vi "HardwareLogLoop.vi"(8 "Error In":errorcluster, 9 "ABLE Configuration":T1, 10 "Hardware Log Data":refnum<queue>, 11 "Hardware Log Action Queue":refnum<queue>) -> (0 "Error Out":errorcluster)   [LabVIEW 2012]
uses:
  ABLEConfiguration.ctl
  DisplayConfiguration.ctl
  FolderConfiguration.ctl
  AlarmsConfiguration.ctl
  Keithley6485Configuration.ctl
  Keithley6482Configuration.ctl
  HardwareLogActionQueueElement.ctl
  HardwareLogAction.ctl
  HardwareLogData.ctl
  HardwareDisplayData.ctl
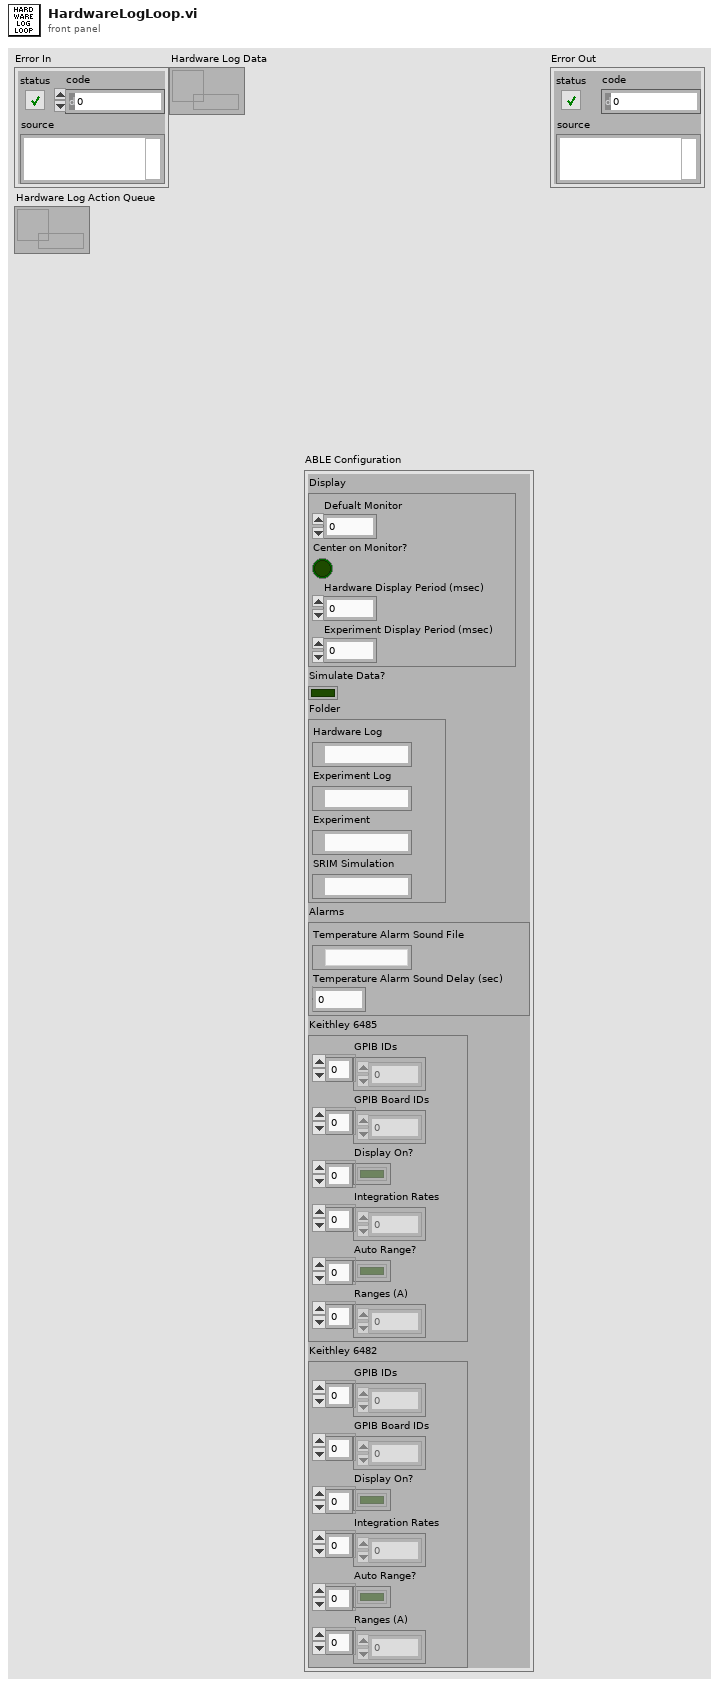
[diagram p1: front panel]
types:
  T1 = typedef "ABLEConfiguration.ctl" = cluster{"Display":T2, "Simulate Data?":bool, "Folder":T3, "Alarms":T4, "Keithley 6485":T5, "Keithley 6482":T6}
  T2 = typedef "DisplayConfiguration.ctl" = cluster{"Defualt Monitor":u16, "Center on Monitor?":bool, "Hardware Display Period (msec)":u32, "Experiment Display Period (msec)":u32}
  T3 = typedef "FolderConfiguration.ctl" = cluster{"Hardware Log":path, "Experiment Log":path, "Experiment":path, "SRIM Simulation":path}
  T4 = typedef "AlarmsConfiguration.ctl" = cluster{"Temperature Alarm Sound File":path, "Temperature Alarm Sound Delay (sec)":dbl}
  T5 = typedef "Keithley6485Configuration.ctl" = cluster{"GPIB IDs":u8[], "GPIB Board IDs":u8[], "Display On?":bool[], "Integration Rates":dbl[], "Auto Range?":bool[], "Ranges (A)":dbl[]}
  T6 = typedef "Keithley6482Configuration.ctl" = cluster{"GPIB IDs":u8[], "GPIB Board IDs":u8[], "Display On?":bool[], "Integration Rates":dbl[], "Auto Range?":bool[], "Ranges (A)":dbl[]}
  T7 = typedef "HardwareLogActionQueueElement.ctl" = cluster{"Action":T8, "Data":variant}
  T8 = typedef "HardwareLogAction.ctl" = enum16{"Initialize", "Clear", "Create", "Log", "Stop", "Shutdown"}
  T9 = enum16{"open", "replace", "create", "open or create", "replace or create", "replace or create with confirmation"}
  T10 = typedef "HardwareLogData.ctl" = cluster{"Time Stamp":timestamp, "Data":T11}
  T11 = typedef "HardwareDisplayData.ctl" = cluster{"Temperatures (C)":dbl[], "Terminal Voltage (MeV)":dbl, "Currents (A)":dbl[]}
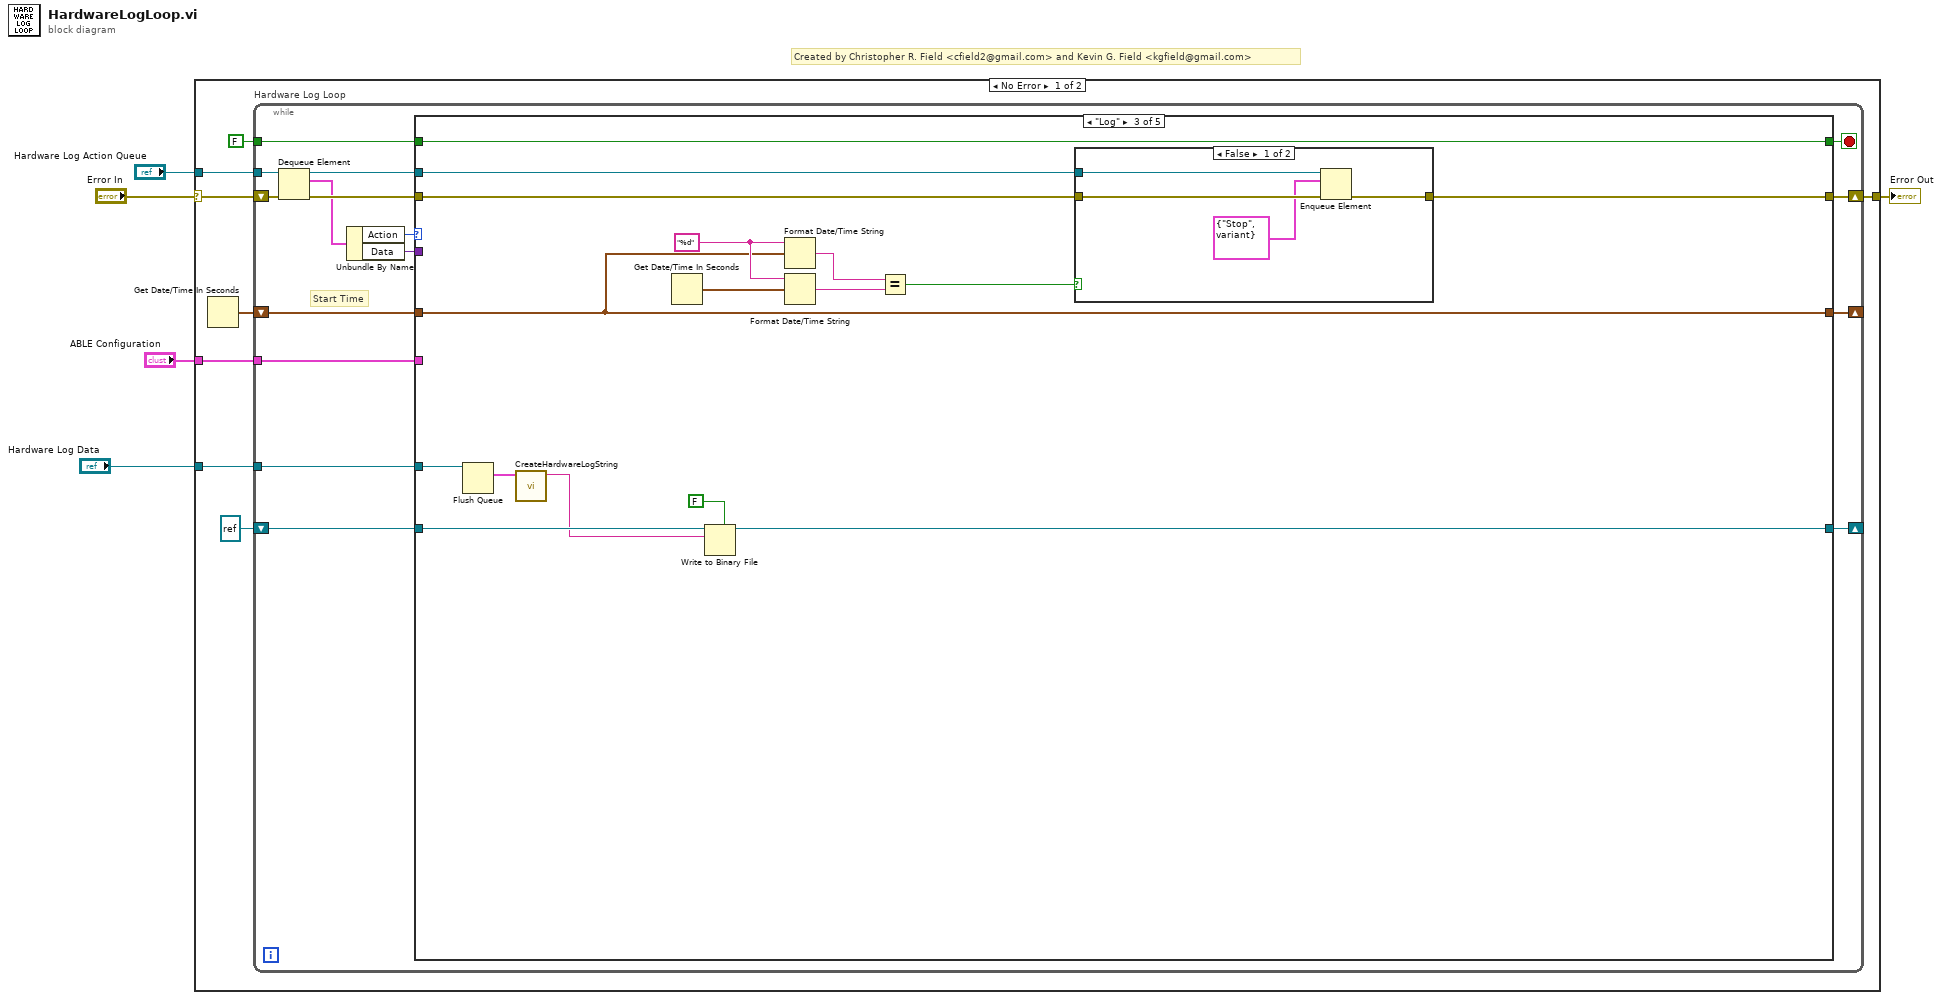
[diagram p0: block diagram]
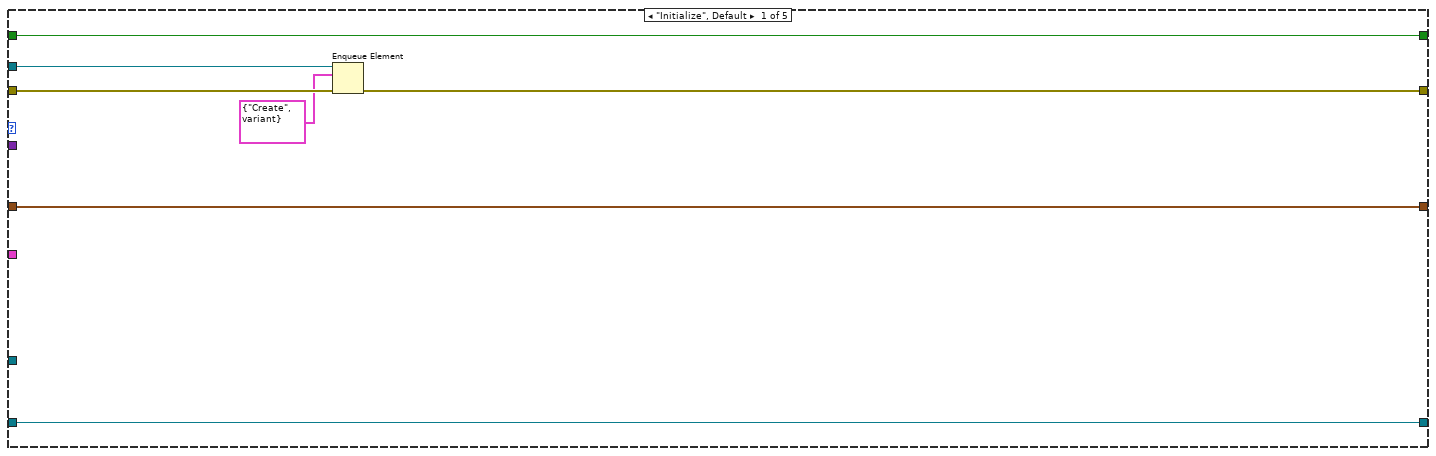
[diagram p2: hidden frame]
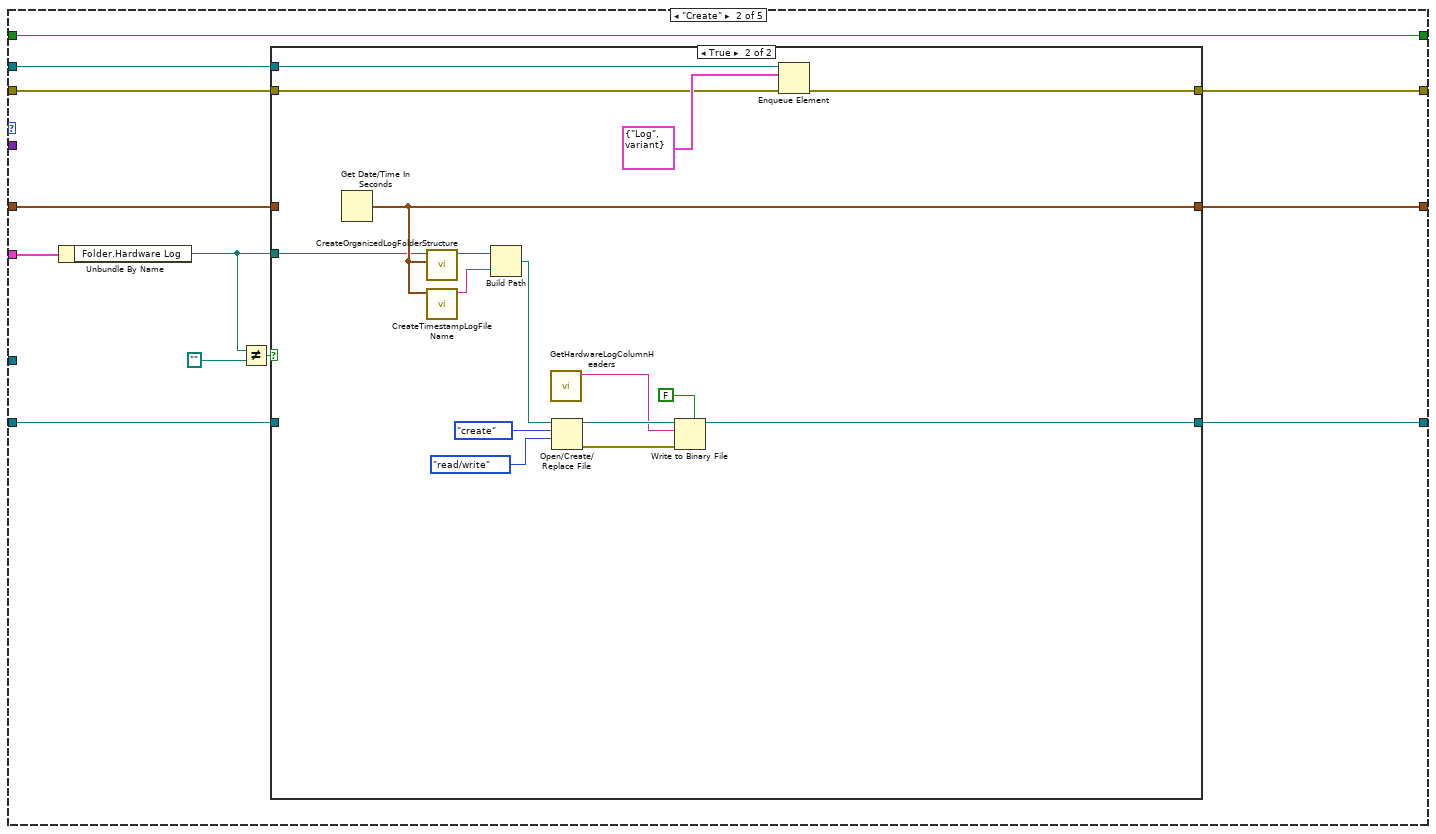
[diagram p3: hidden frame]
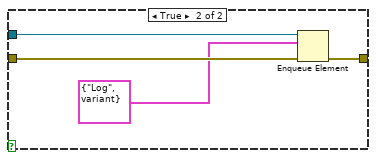
[diagram p5: hidden frame]
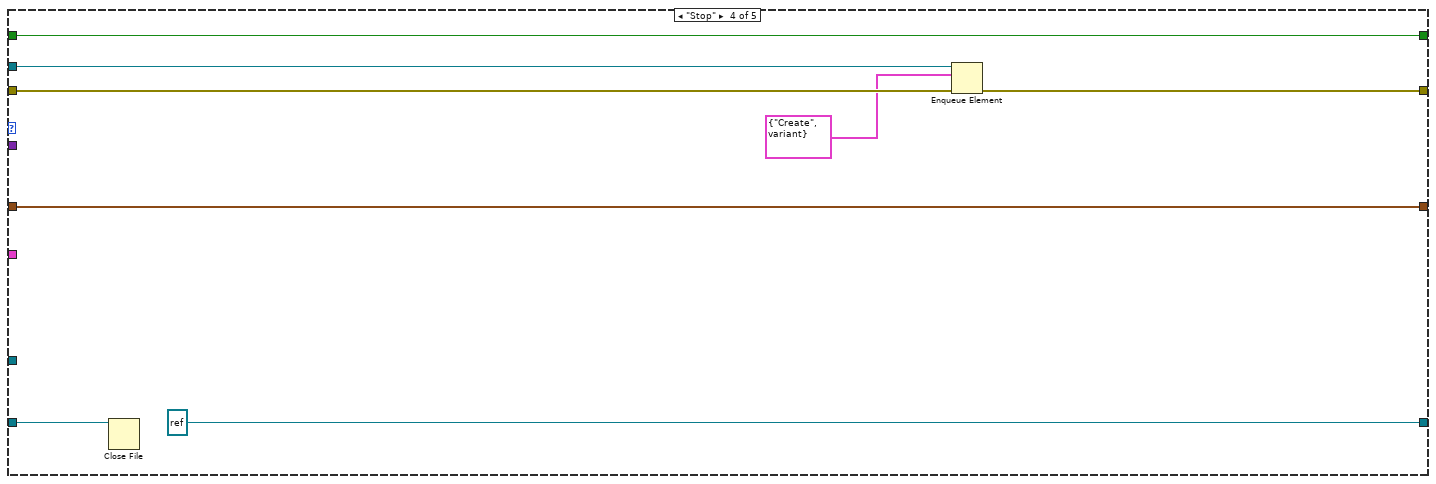
[diagram p6: hidden frame]
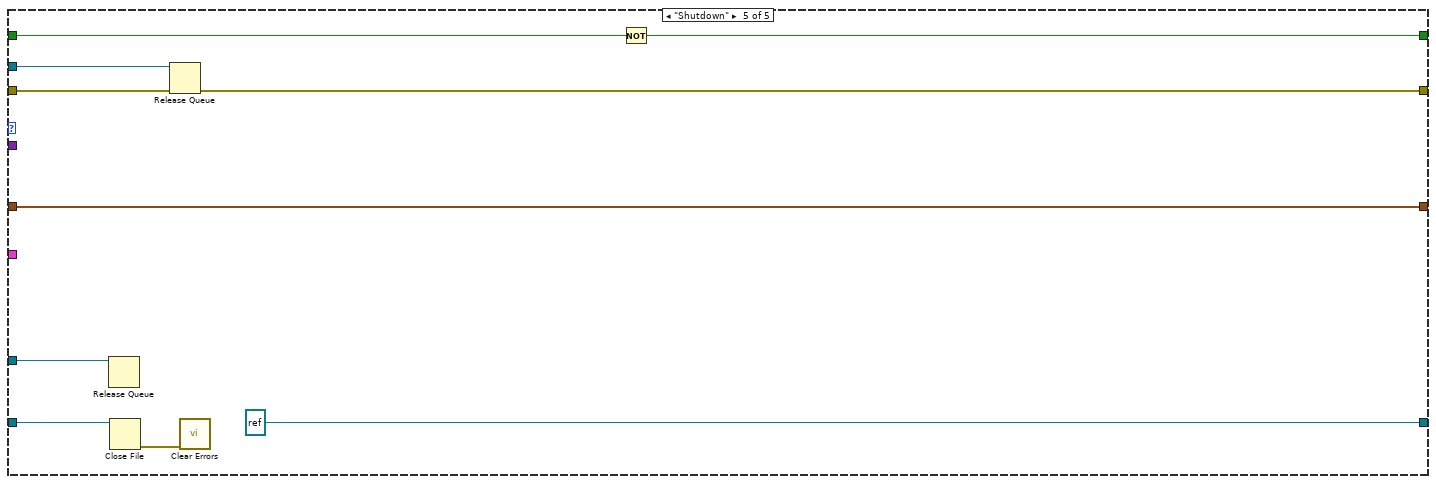
[diagram p7: hidden frame]
diagram:
  # "Created by Christopher R. Field <cfield2@gmail.com> and Kevin G. Field <kgfield@gmail.com>"
  n1 = case shown="No Error" "Error In" {
    selector: "Error In" -> [w12 w110]
    tunnel: [w11 w110] -> w5
    tunnel: "ABLE Configuration" -> [w8 _]
    tunnel: "Hardware Log Action Queue" -> [w10 _]
    tunnel: "Hardware Log Data" -> [w9 _]
    frame No Error {
      n2 = Get Date/Time In Seconds() -> (seconds since 1Jan1904=w6:timestamp)
      n3 = while "Hardware Log Loop" {
        tunnel: FALSE -> [w29]
        shift-right: [w26] -> w11
        shift-left: w12 -> [w28]
        tunnel: w10 -> [w20]
        tunnel: w9 -> [w19]
        tunnel: w8 -> [w18]
        shift-right: [w17] -> _
        shift-left: refnum<file> refnum ("refnum out") -> [w16]
        shift-right: [w15] -> _
        shift-left: w6 -> [w14]
        stop <- w21 stop-if-true
        # "Start Time"
        n4 = Dequeue Element(queue=w20, error in (no error)=w28) -> (queue out=w22:refnum<queue>, element=w25:T7, error out=w27:errorcluster)  [unwired: 1 in, 1 out]
        n5 = Unbundle By Name(w25) -> ("Action"=w24:T8, "Data"=w23:variant)
        n6 = case shown="\"Log\"" w24 {
          tunnel: w29 -> [w36 w48 w83 w96 w109]
          tunnel: w27 -> [w34 w38 w69 w98 w105]
          tunnel: [w33 w39 w68 w97 w104] -> w26
          tunnel: w23 -> [_ _ _ _ _]
          tunnel: w22 -> [w35 w40 w70 w99 w106]
          tunnel: [w36 w48 w83 w96 w108] -> w21
          tunnel: w19 -> [_ _ w77 _ w107]
          tunnel: w18 -> [_ w47 _ _ _]
          tunnel: [w30 w44 w72 refnum<file> refnum ("refnum out") refnum<file> refnum ("refnum out")] -> w17
          tunnel: w16 -> [w30 w43 w75 w94 w102]
          tunnel: [w31 w42 w78 w92 w103] -> w15
          tunnel: w14 -> [w31 w41 w78 w92 w103]
          frame "Initialize", Default {
            n7 = Enqueue Element(queue=w35, element=T7 {"Action"=enum."Create", "Data"=variant}, error in (no error)=w34) -> (error out=w33:errorcluster)  [unwired: 1 in, 2 out]
          }
          frame "Create" {
            n8 = Unbundle By Name(w47) -> ("Folder.Hardware Log"=w45:path)
            n9 = Not Equal?(x=w45, y=path "") -> (x != y?=w37:bool)
            n10 = case shown="True" w37 {
              tunnel: w45 -> [_ w52]
              tunnel: [w51 w62] -> w44
              tunnel: w43 -> [w51 _]
              tunnel: [w50 w58] -> w42
              tunnel: w41 -> [w50 _]
              tunnel: w40 -> [_ w55]
              tunnel: [w49 w54] -> w39
              tunnel: w38 -> [w49 w53]
              frame False {
              }
              frame True {
                n11 = Get Date/Time In Seconds() -> (seconds since 1Jan1904=w58:timestamp)
                n12 = call "CreateOrganizedLogFolderStructure.vi"("Time Stamp"=w58, "Base Log Path"=w52) -> ("Organized Log Path"=w59:path)  [unwired: 8 in, 1 out]
                n13 = call "CreateTimestampLogFileName.vi"("Time Stamp"=w58) -> ("Timestamp Log File Name"=w57:string)  [unwired: 10 in]
                n14 = Build Path(base path=w59, name or relative path=w57) -> (appended path=w67:path)
                n15 = call "GetHardwareLogColumnHeaders.vi"() -> ("Column Headers"=w61:string)  [unwired: 11 in]
                n16 = Open/Create/Replace File(file path (use dialog)=w67, operation (0:open)=T9."create", access (0:read/write)=enum16{"read/write", "read-only", "write-only"}."read/write") -> (refnum out=w64:refnum<file>, error out=w63:errorcluster)  [unwired: 3 in, 1 out]
                n17 = Write to Binary File(file (use dialog)=w64, data=w61, error in=w63, 5:FALSE ("prepend array or string size? (T)")) -> (refnum out=w62:refnum<file>)  [unwired: 2 in, 2 out]
                n18 = Enqueue Element(queue=w55, element=T7 {"Action"=enum."Log", "Data"=variant}, error in (no error)=w53) -> (error out=w54:errorcluster)  [unwired: 1 in, 2 out]
              }
            }
          }
          frame "Log" {
            w81 = "%d" ("time format string (%c)")
            n19 = Flush Queue(queue=w77) -> (remaining elements=w76:T10[])  [unwired: 1 in, 2 out]
            n20 = call "CreateHardwareLogString.vi"("Hardware Log Data Queue Elements"=w76) -> ("Hardware Log String"=w74:string)  [unwired: 10 in]
            n21 = Get Date/Time In Seconds() -> (seconds since 1Jan1904=w82:timestamp)
            n22 = Write to Binary File(file (use dialog)=w75, data=w74, 5:FALSE ("prepend array or string size? (T)")) -> (refnum out=w72:refnum<file>)  [unwired: 3 in, 2 out]
            n23 = Format Date/Time String(time format string (%c)=w81, seconds (now)=w78) -> (date/time string=w80:string)  [unwired: 1 in]
            n24 = Format Date/Time String(time format string (%c)=w81, seconds (now)=w82) -> (date/time string=w79:string)  [unwired: 1 in]
            n25 = Equal?(x=w80, y=w79) -> (x = y?=w71:bool)
            n26 = case shown="False" w71 {
              tunnel: w70 -> [w87 w91]
              tunnel: w69 -> [w86 w90]
              tunnel: [w84 w89] -> w68
              frame False {
                n27 = Enqueue Element(queue=w87, element=T7 {"Action"=enum."Stop", "Data"=variant}, error in (no error)=w86) -> (error out=w84:errorcluster)  [unwired: 1 in, 2 out]
              }
              frame True {
                n28 = Enqueue Element(queue=w91, element=T7 {"Action"=enum."Log", "Data"=variant}, error in (no error)=w90) -> (error out=w89:errorcluster)  [unwired: 1 in, 2 out]
              }
            }
          }
          frame "Stop" {
            n29 = Close File(refnum=w94) -> ()  [unwired: 1 in, 2 out]
            n30 = Enqueue Element(queue=w99, element=T7 {"Action"=enum."Create", "Data"=variant}, error in (no error)=w98) -> (error out=w97:errorcluster)  [unwired: 1 in, 2 out]
          }
          frame "Shutdown" {
            n31 = Release Queue(queue=w107) -> ()  [unwired: 2 in, 3 out]
            n32 = Close File(refnum=w102) -> (error out=w100:errorcluster)  [unwired: 1 in, 1 out]
            n33 = Release Queue(queue=w106, error in (no error)=w105) -> (error out=w104:errorcluster)  [unwired: 1 in, 2 out]
            n34 = call <vilib>:"Clear Errors.vi"("error in (no error)"=w100) -> ()  [unwired: 6 in, 1 out]
            n35 = Not(x=w109) -> (.not. x?=w108:bool)
          }
        }
      }
    }
    frame Error {
    }
  }
  "Error Out" <- w5
